vi "lesker.vi"() -> ()   [LabVIEW 2012]
panel:
  out "Pressure (Torr)":dbl
  in  "stop":bool
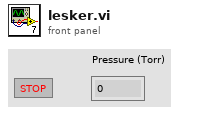
[diagram p1: front panel]
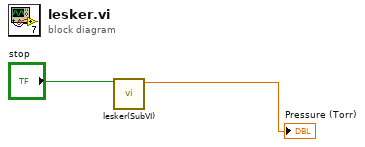
[diagram p0: block diagram]
diagram:
  n1 = call "lesker(SubVI).vi"("stop"="stop") -> ("Pressure (Torr)"=→"Pressure (Torr)":dbl)  [unwired: 10 in]
